vi "drop_handle.vi"(0 "Message":T1) -> (1 "error out":errorcluster, 2 "drop-array":string[](array[string]), 3 "file count":u32)   [LabVIEW 2012]
uses:
  shell32.dll
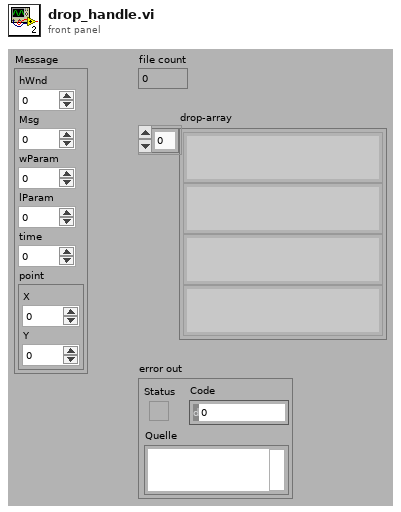
[diagram p1: front panel]
types:
  T1 = cluster{"hWnd":u32, "Msg":u32, "wParam":u32, "lParam":i32, "time":u32, "point":cluster{"X":i32, "Y":i32}}
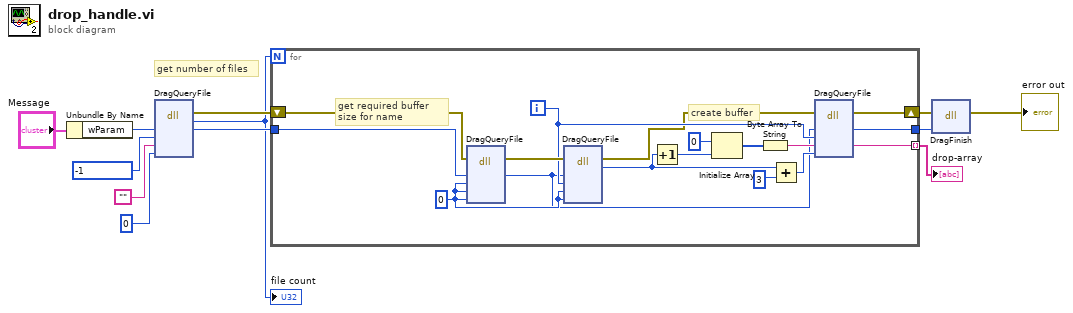
[diagram p0: block diagram]
diagram:
  # "get number of files"
  n1 = Unbundle By Name("Message") -> ("wParam"=w1:u32)
  n2 = dll-call lib="shell32.dll" fn="DragQueryFile"("hDrop"=w1, "iFile"=-1, "lpszFile"="", "cch"=0) -> (error out=w4:errorcluster, "return type"=w3:u32, "hDrop"=w5:i32)  [unwired: 6 in, 1 out]
  "file count" <- w3
  n3 = for {
    N: w3 -> [_]
    shift-right: [w24] -> w6
    shift-left: w4 -> [w16]
    tunnel: w5 -> [w17]
    tunnel: [w25] -> w7
    tunnel: [w23] -> w11 mode=indexing
    i -> [w18]
    w20 = 0
    # "create buffer"
    # "get required buffer size for name"
    n4 = dll-call lib="shell32.dll" fn="DragQueryFile"(error in=w16, "hDrop"=w17, "iFile"=w20, "lpszFile"=w20, "cch"=w20) -> (error out=w19:errorcluster, "hDrop"=w13:i32)  [unwired: 6 in, 1 out]
    n5 = dll-call lib="shell32.dll" fn="DragQueryFile"(error in=w19, "hDrop"=w13, "iFile"=w18, "lpszFile"=w20, "cch"=w20) -> (error out=w15:errorcluster, "return type"=w14:u32)  [unwired: 6 in, 1 out]
    n6 = Increment(x=w14) -> (x+1=w27:u32)
    n7 = Initialize Array(u8 0, w27) -> (w29:u8[])
    n8 = Byte Array To String(unsigned byte array=w29) -> (string=w26:string)
    n9 = Add(x=w14, y=u32 3) -> (x+y=w21:u32)
    n10 = dll-call lib="shell32.dll" fn="DragQueryFile"(error in=w15, "hDrop"=w13, "iFile"=w18, "lpszFile"=w26, "cch"=w21) -> (error out=w24:errorcluster, "hDrop"=w25:i32, "lpszFile"=w23:string)  [unwired: 5 in, 1 out]
  }
  "drop-array" <- w11
  n11 = dll-call lib="shell32.dll" fn="DragFinish"(error in=w6, "hDrop"=w7) -> (error out=→"error out":errorcluster)  [unwired: 4 in, 1 out]
